vi "Set FirstContactFlags.vi"(8 "Limits Cluster in":cluster{"flow":dbl[], "temp":dbl[]}, 9 "nr iterations delay":u8=1, 10 "iteration in":u8, 11 "first flags in":T1) -> (2 "iteration out":u8, 3 "first flags out":T1)   [LabVIEW 2020, in "Linearisierung v2.lvlib" / "Gasteiler.lvlib" / "HovaCAL_Interface.lvlib" / "Kommunikation.lvlib"]
uses:
  Kommunikation.lvlib
  Aktion_FGV_HovaCAL_Interface_GetData.ctl
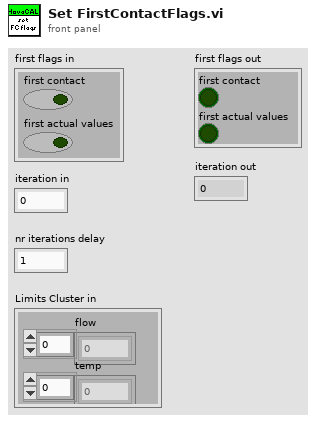
[diagram p1: front panel]
types:
  T1 = cluster{"first contact":bool, "first actual values ":bool}
  T2 = typedef "Linearisierung v2.lvlib/Gasteiler.lvlib/HovaCAL_Interface.lvlib/Kommunikation.lvlib/Aktion_FGV_HovaCAL_Interface_GetData.ctl" = enum16{"lesen", "SystemInfo", "MFC Info", "actual Values", "Limits", "first contact"}
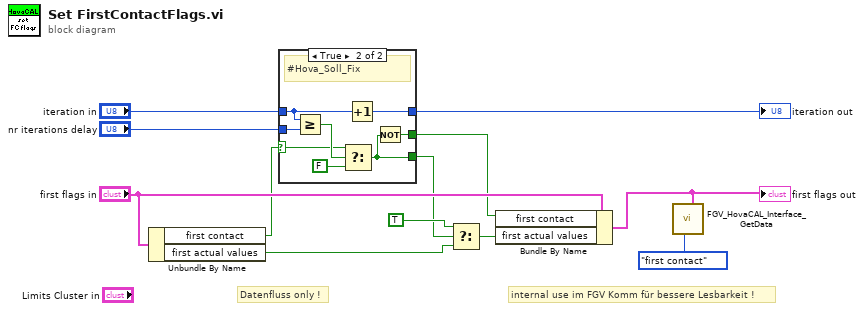
[diagram p0: block diagram]
diagram:
  # "internal use im FGV Komm für bessere Lesbarkeit !"
  # "Datenfluss only !"
  n1 = Unbundle By Name("first flags in") -> ("first contact"=w6:bool, "first actual values"=w7:bool)
  n2 = case shown="True" w6 {
    selector: w6 -> [_ w16]
    tunnel: "iteration in" -> [_ w19]
    tunnel: [_ w20] -> w4
    tunnel: "nr iterations delay" -> [_ w18]
    tunnel: [_ w14] -> w2
    tunnel: [_ w13] -> w1
    frame False {
    }
    frame True {
      # "#Hova_Soll_Fix"
      n3 = Greater Or Equal?(x=w19, y=w18) -> (x >= y?=w17:bool)
      n4 = Select(t=w16, s=w17, f=FALSE) -> (s? t:f=w14:bool)
      n5 = Increment(x=w19) -> (x+1=w20:u8)
      n6 = Not(x=w14) -> (.not. x?=w13:bool)
    }
  }
  "iteration out" <- w4
  n7 = Select(t=TRUE, s=w2, f=w7) -> (s? t:f=w10:bool)
  n8 = Bundle By Name(cluster="first flags in", "first contact"=w1, "first actual values"=w10) -> (w12:T1)
  "first flags out" <- w12
  n9 = call "FGV_HovaCAL_Interface_GetData.vi"("first flags in"=w12, "Aktion"=Aktion_FGV_HovaCAL_Interface_GetData."first contact") -> ()  [unwired: 5 in, 5 out]
